vi "全局 1.vi"() -> ()   [LabVIEW 2018]
panel:
  in  "选项卡控件":T1(tab)
  out "Login":bool
  out "Login PW":dbl=12.34 format="%.2f"
  out "CCIEFB Slave IP":string="192.168.2.100"
  out "ROBOT PORT":u16 format="%08x"
  out "ROBOT IP":string
  out "PLC PORT":u16 format="%08x"
  out "PLC IP":string
  out "ini文件":path
  out "产品名称":string
  out "Exit":bool
  in  "拨钮上下Pr":T2={"选择"=enum."Fx", "系数"=1.0, "上限"=2.55, "下限"=2.05, "Ymax"=5.0, "Ymin"=-5.0, "点数"=1000.0, "起点"=0.0, "终点"=0.0} {"终点" format="%.2f"; "起点" format="%.2f"; "下限" format="%.2f"; "上限" format="%.2f"; "系数" format="%.3f"}
  in  "拨钮下上Pr":T2={"选择"=enum."Fx", "系数"=1.0, "上限"=2.55, "下限"=2.05, "Ymax"=5.0, "Ymin"=-5.0, "点数"=1000.0, "起点"=0.0, "终点"=0.0} {"终点" format="%.2f"; "起点" format="%.2f"; "下限" format="%.2f"; "上限" format="%.2f"; "系数" format="%.3f"}
  in  "拨钮左右Pr":T2={"选择"=enum."Fx", "系数"=1.0, "上限"=2.55, "下限"=2.05, "Ymax"=5.0, "Ymin"=-5.0, "点数"=1000.0, "起点"=0.0, "终点"=0.0} {"终点" format="%.2f"; "起点" format="%.2f"; "下限" format="%.2f"; "上限" format="%.2f"; "系数" format="%.3f"}
  in  "拨钮右左Pr":T2={"选择"=enum."Fx", "系数"=1.0, "上限"=2.55, "下限"=2.05, "Ymax"=5.0, "Ymin"=-5.0, "点数"=1000.0, "起点"=0.0, "终点"=0.0} {"终点" format="%.2f"; "起点" format="%.2f"; "下限" format="%.2f"; "上限" format="%.2f"; "系数" format="%.3f"}
  in  "轮盘开关Pr":T3={"选择"=enum."Fx", "系数"=1.0, "上限"=4.3, "下限"=3.7, "Ymax"=50.0, "Ymin"=-50.0, "点数"=1000.0, "锁系数x"=1.0, "锁上限"=0.4, "锁下限"=0.6, "锁系数+"=1.0, "起点"=0.20000000298023224, "终点"=0.6499999761581421, "锁起点"=0.05000000074505806, "锁终点"=0.20000000298023224} {"锁终点" format="%.2f"; "锁起点" format="%.2f"; "终点" format="%.2f"; "起点" format="%.2f"; "锁系数+" format="%.3f"; "锁下限" format="%.2f"; "锁上限" format="%.2f"; "锁系数x" format="%.3f"; "下限" format="%.2f"; "上限" format="%.2f"; "系数" format="%.3f"}
  in  "轮盘关开Pr":T3={"选择"=enum."Fx", "系数"=1.0, "上限"=4.3, "下限"=3.7, "Ymax"=50.0, "Ymin"=-50.0, "点数"=1000.0, "锁系数x"=1.0, "锁上限"=0.4, "锁下限"=0.6, "锁系数+"=1.0, "起点"=0.20000000298023224, "终点"=0.6499999761581421, "锁起点"=0.05000000074505806, "锁终点"=0.20000000298023224} {"锁终点" format="%.2f"; "锁起点" format="%.2f"; "终点" format="%.2f"; "起点" format="%.2f"; "锁系数+" format="%.3f"; "锁下限" format="%.2f"; "锁上限" format="%.2f"; "锁系数x" format="%.3f"; "下限" format="%.2f"; "上限" format="%.2f"; "系数" format="%.3f"}
  out "拨钮下上力检":cluster{"判断完成":bool, "不合格?":bool}
  out "拨钮上下力检":cluster{"判断完成":bool, "不合格?":bool}
  out "拨钮右左力检":cluster{"判断完成":bool, "不合格?":bool}
  out "拨钮左右力检":cluster{"判断完成":bool, "不合格?":bool}
  out "轮盘开关力检":cluster{"判断完成":bool, "不合格?":bool}
  out "轮盘关开力检":cluster{"判断完成":bool, "不合格?":bool}
  out "PC状态":cluster{"PLC就绪":bool, "空动作中":bool}
  out "PLC结果":T4
  out "PLC状态":T5
  out "力":sgl[](array[numeric]) format="%.2f"
  out "检测步骤":T6
  out "PLC检测值":T7 {"LED电压" format="%.2f"; "LED电流" format="%.1f"; "风门开电压" format="%.2f"; "风门闭电压" format="%.2f"; "稳定压力" format="%.1f"; "当前压力" format="%.1f"; "稳定泄漏量" format="%.2f"; "当前泄漏量" format="%.2f"}
  out "高低配":i16
  out "PLC检测参数":T8 {"伺服速度" format="%.1f"; "气压稳定时间" format="%.1f"; "LED电流下限" format="%.1f"; "LED电流上限" format="%.1f"; "风门开电压下限" format="%.2f"; "风门开电压上限" format="%.2f"; "风门闭电压下限" format="%.2f"; "风门闭电压上限" format="%.2f"; "压力下限" format="%.1f"; "压力上限" format="%.1f"; "泄漏量上限" format="%.2f"; "轮盘预压力" format="%.1f"}
  out "RX":bool[][](array[boolean])
  in  "RWr":i16[][](array[numeric]) format="%04x"
  out "视觉检测":u16[](array[numeric])
  out "SQL_Data":T9
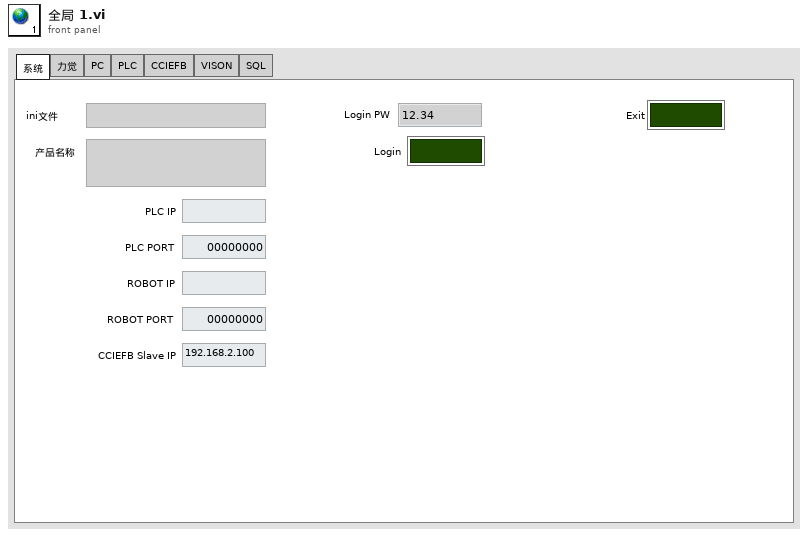
[diagram p1: front panel]
types:
  T1 = enum32{"系统", "力觉", "PC", "PLC", "CCIEFB", "VISON", "SQL"}
  T2 = cluster{"选择":enum16{"Fx", "Fy", "Fz", "Mx", "My", "Mz"}, "系数":sgl, "上限":sgl, "下限":sgl, "Ymax":dbl, "Ymin":dbl, "点数":dbl, "起点":dbl, "终点":dbl}
  T3 = cluster{"选择":enum16{"Fx", "Fy", "Fz", "Mx", "My", "Mz"}, "系数":sgl, "上限":sgl, "下限":sgl, "Ymax":dbl, "Ymin":dbl, "点数":dbl, "锁系数x":sgl, "锁上限":sgl, "锁下限":sgl, "锁系数+":sgl, "起点":dbl, "终点":dbl, "锁起点":dbl, "锁终点":dbl}
  T4 = cluster{"泄漏量":bool, "风门闭电压":bool, "风门开电压":bool, "LED电压":bool, "LED电流":bool, "拍照1":bool, "拍照2":bool, "拍照3":bool}
  T5 = cluster{"PLC就绪":bool, "ROBOT就绪":bool, "空动作":bool, "检测NG":bool, "检测结束":bool, "检测开始":bool, "初始化脉冲":bool}
  T6 = cluster{"泄漏量":bool, "风门开闭电检":bool, "LED电检":bool, "拍照位1":bool, "拍照位2":bool, "拍照位3":bool, "轮盘关开":bool, "轮盘关开锁":bool, "轮盘开关":bool, "轮盘开关锁":bool, "拨钮左右":bool, "拨钮右左":bool, "拨钮上下":bool, "拨钮下上":bool}
  T7 = cluster{"当前泄漏量":sgl, "稳定泄漏量":sgl, "当前压力":sgl, "稳定压力":sgl, "风门闭电压":sgl, "风门开电压":sgl, "LED电流":sgl, "LED电压":sgl}
  T8 = cluster{"轮盘预压力":sgl, "泄漏量上限":sgl, "压力上限":sgl, "压力下限":sgl, "风门闭电压上限":sgl, "风门闭电压下限":sgl, "风门开电压上限":sgl, "风门开电压下限":sgl, "LED电流上限":sgl, "LED电流下限":sgl, "气压稳定时间":sgl, "伺服速度":sgl}
  T9 = cluster{"cMacCode":string, "cInvCode":string, "cCheckDate":timestamp, "cCheckNo":string, "cState":string, "cDefine1":string, "cDefine2":string, "cDefine3":string, "cDefine4":string, "cDefine5":string, "cDefine6":string, "cDefine7":string, "cDefine8":string, "cDefine9":string, "cDefine10":string, "cDefine11":string, "cDefine12":string, "cDefine13":string, "cDefine14":string, "cDefine15":string, "cDefine16":string, "cDefine17":string, "cDefine18":string}
diagram:
